vi "Read Key.vi"(6 "Key":string, 8 "error in (no error)":errorcluster, 11 "Configuration in":refnum<class "Configuration.lvclass">) -> (0 "error out":errorcluster, 2 "Value":string, 3 "Configuration out":refnum<class "Configuration.lvclass">)   [LabVIEW 2023, in "Configuration.lvlib" / "Configuration.lvclass"]
doc: "This routine searches the configuration defintion for the ancestor class' defintion file, accesses the key by name and returns the key's value. \n\n<b>Inputs</b>\nString <b>Key</b> - This is the specific key the ancestor class is requesting\n\n<b>Outputs</b>\nString <b>Value</b> - This is the specific value associated with the ancestor class' configuration item"
uses:
  Library/Configuration.lvclass
  Library/Configuration.lvclass/Configuration.ctl
  builds/Framework/Actor Framework.lvlibp/1abvi3w/vi.lib/ActorFramework/Actor/Read Actor Label.vi
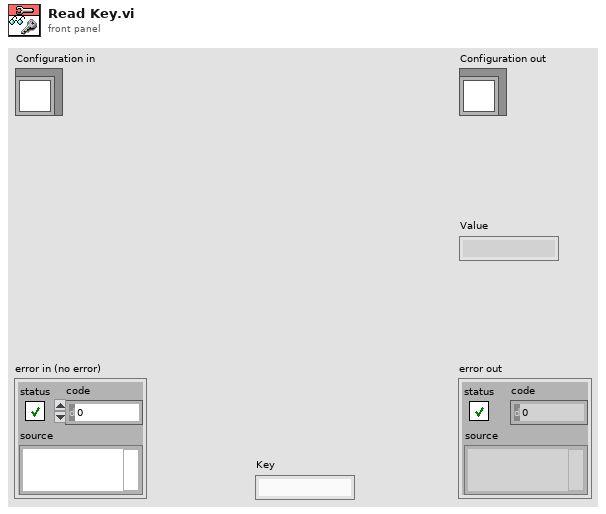
[diagram p1: front panel]
types:
  T1 = typedef "Configuration.lvlib/Configuration.lvclass/Definitions.ctl" = map{string, T2}
  T2 = typedef "Configuration.lvlib/Configuration.lvclass/Config.ctl" = map{string, string}
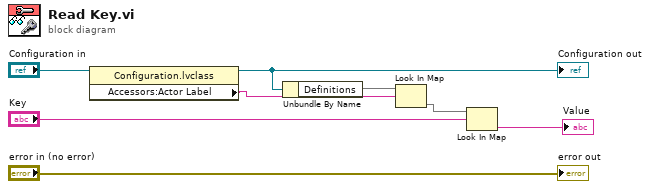
[diagram p0: block diagram]
diagram:
  n1 = property class="Configuration.lvclass"(reference="Configuration in") -> (reference out=w2:refnum<class "Configuration.lvclass">, "Accessors:Actor Label"=w3:string)  [unwired: 1 in, 1 out]
  "Configuration out" <- w2
  n2 = Unbundle By Name(w2) -> ("Definitions"=w7:T1)
  n3 = Look In Map(map=w7, key=w3) -> (value=w6:T2)  [unwired: 1 in, 1 out]
  n4 = Look In Map(map=w6, key="Key") -> (value=→"Value":string)  [unwired: 1 in, 1 out]
  "error out" <- "error in (no error)"
